vi "Get Queue Names.vi"(11 "Queue references":T1[](array[typedef])) -> (3 "Queue Names":string[](array[string]))   [LabVIEW 2013, in "Interloop MessageQ.lvlib"]
uses:
  Interloop MessageQ.lvlib
  Message Queue Ref.ctl
  Message cluster.ctl
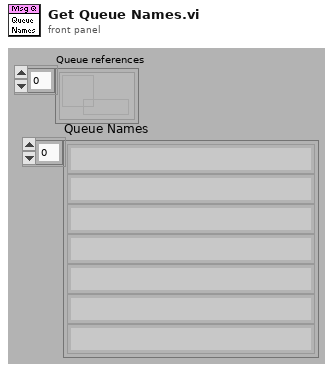
[diagram p1: front panel]
types:
  T1 = typedef "Interloop MessageQ.lvlib/Message Queue Ref.ctl" = refnum<queue>
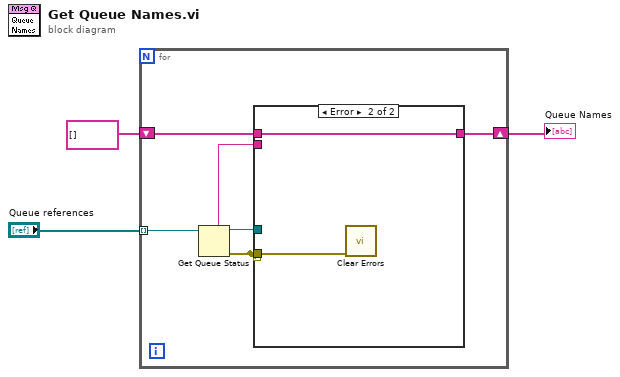
[diagram p0: block diagram]
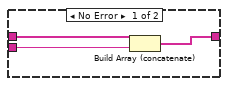
[diagram p2: hidden frame]
diagram:
  n1 = for {
    tunnel: "Queue references" -> [w9] mode=indexing
    shift-right: [w5] -> w3
    shift-left: string[] [] ("Queue Names") -> [w6]
    n2 = Get Queue Status(queue=w9) -> (queue out=w8:T1, queue name=w4:string, error out=w7:errorcluster)  [unwired: 1 in, 6 out]
    n3 = case shown="Error" w7 {
      tunnel: w8 -> [_ _]
      tunnel: w7 -> [_ w14]
      tunnel: w6 -> [w12 w13]
      tunnel: [w10 w13] -> w5
      tunnel: w4 -> [w11 _]
      frame No Error {
        n4 = Build Array (concatenate)(w12, w11) -> (w10:string[])
      }
      frame Error {
        n5 = call <vilib>:"Clear Errors.vi"("error in (no error)"=w14) -> ()  [unwired: 7 out]
      }
    }
  }
  "Queue Names" <- w3
